vi "Interface_GetReference_4x4x4.vi"(8 "error in (no error)":errorcluster, 11 "reference in":refnum<class>) -> (0 "error out":errorcluster, 2 "InterfaceOut":refnum<class>, 3 "reference out":refnum<class>)   [LabVIEW 2010]
doc: "Returns an Interaface that this class implements"
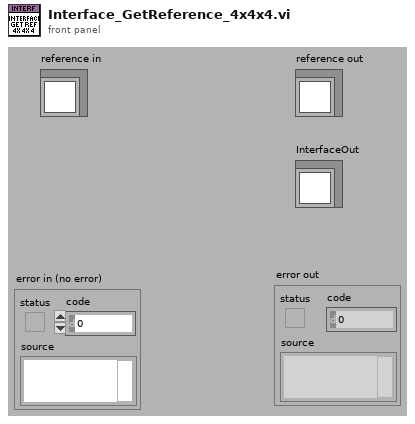
[diagram p1: front panel]
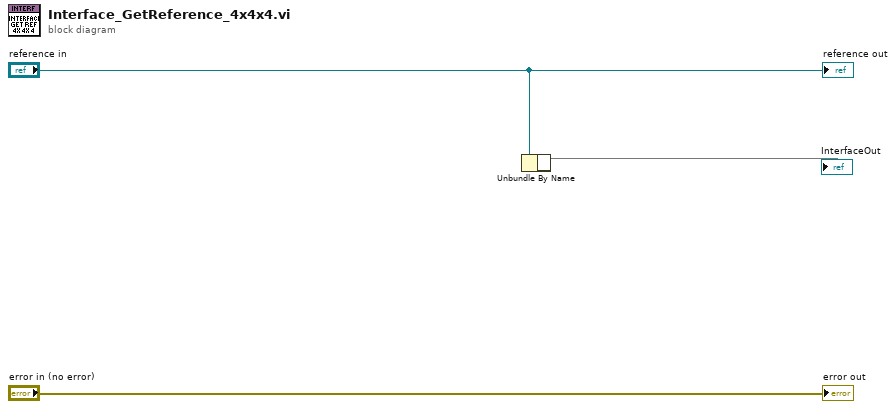
[diagram p0: block diagram]
diagram:
  n1 = Unbundle By Name("reference in") -> (→"InterfaceOut")
  "error out" <- "error in (no error)"
  "reference out" <- "reference in"
